vi "EQC merge1Chip.vi"(9 "EQ Leak# folder paths":path[](array[path]), 11 "ChipID":string) -> (0 "Error tick":bool, 1 "quants GOOD":u8, 2 "Merged report":string, 3 "Merged PixelReg":u32[](array[numeric]) format="%.0x")   [LabVIEW 2015, in "VIPM2.lvlib"]
uses:
  VIPM2.lvlib
panel:
  # "If X, some error while\nreading the files"
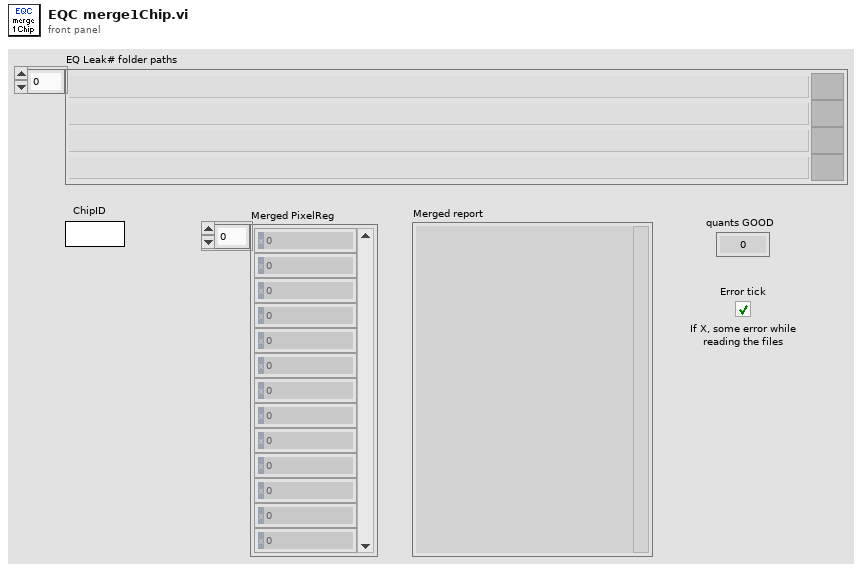
[diagram p1: front panel]
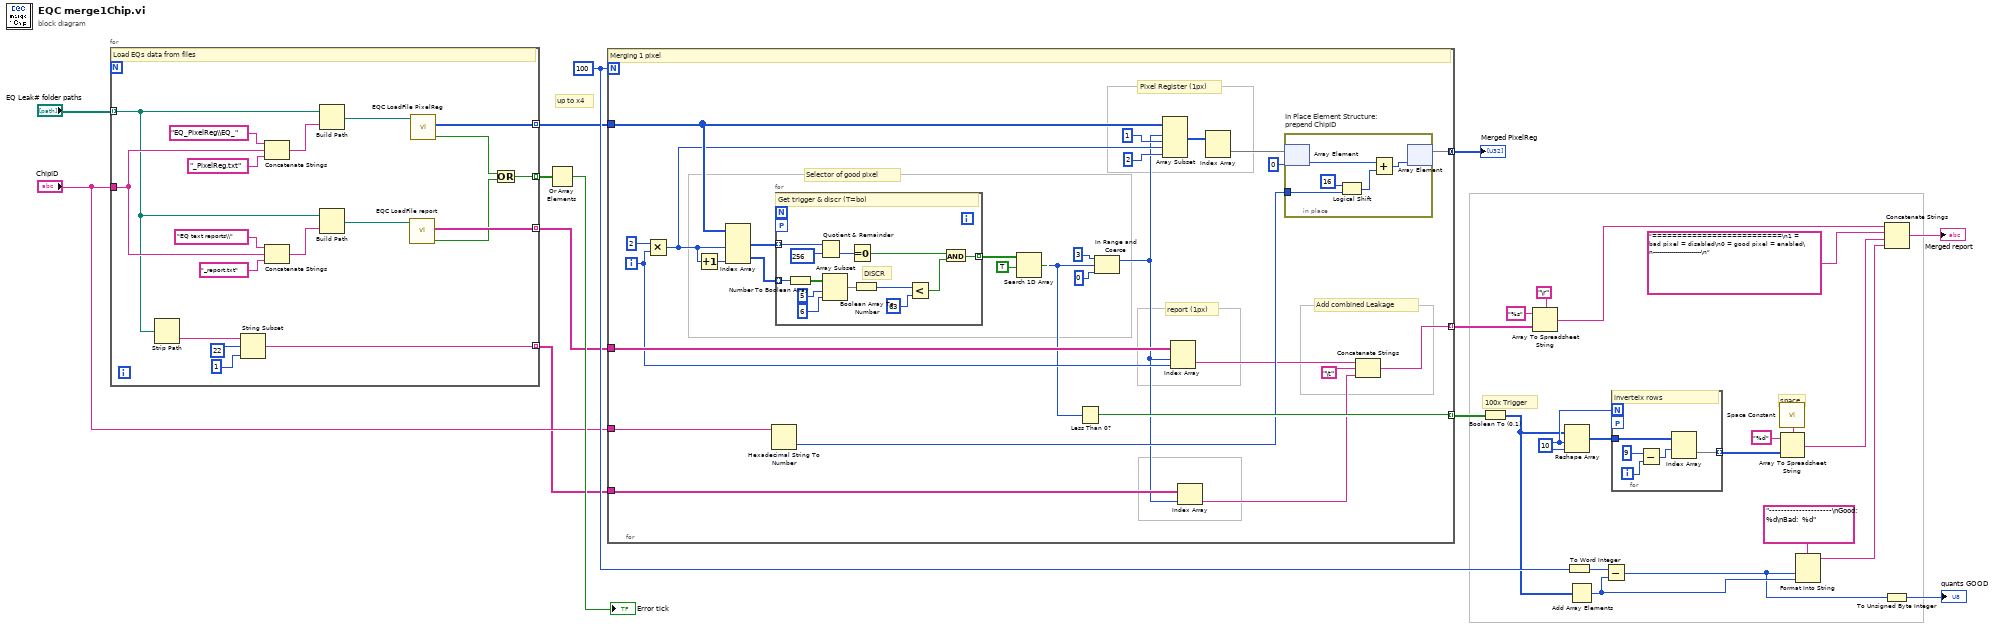
[diagram p0: block diagram]
diagram:
  w13 = 10 ("dimension size")
  w29 = 100
  # "space"
  # "100x Trigger"
  # "up to x4"
  n1 = for {
    tunnel: "EQ Leak# folder paths" -> [w34] mode=indexing
    tunnel: "ChipID" -> [w41]
    tunnel: [w39] -> w25 mode=indexing
    tunnel: [w37] -> w24 mode=indexing
    tunnel: [w35] -> w26 mode=indexing
    tunnel: [w30] -> w1 mode=indexing
    # "Load EQs data from files"
    n2 = Strip Path(path=w34) -> (name=w33:string)  [unwired: 1 out]
    n3 = String Subset(string=w33, offset (0)=22 ("offset"), length (rest)=1 ("length (rest)")) -> (substring=w30:string)
    n4 = Concatenate Strings("EQ_PixelReg\\EQ_", w41, "_PixelReg.txt") -> (w46:string)
    n5 = Concatenate Strings("EQ text reports\\", w41, "_report.txt") -> (w44:string)
    n6 = Build Path(base path=w34, name or relative path=w46) -> (appended path=w45:path)
    n7 = Build Path(base path=w34, name or relative path=w44) -> (appended path=w40:path)
    n8 = call "EQC LoadFile report.vi"("report file path"=w40) -> ("Error tick"=w36:bool, "report (1D lines)"=w37:string[])  [unwired: 9 in]
    n9 = call "EQC LoadFile PixelReg.vi"("PixelReg file path"=w45) -> ("Error tick"=w38:bool, "PixelReg (hex)"=w39:u32[])  [unwired: 9 in]
    n10 = Or(x=w38, y=w36) -> (x .or. y?=w35:bool)
  }
  n11 = Or Array Elements(Boolean array=w26) -> (logical OR=→"Error tick":bool)
  n12 = for {
    N: w29 -> [_]
    tunnel: w25 -> [w70]
    tunnel: w24 -> [w66]
    tunnel: [w61] -> w23 mode=concatenating
    tunnel: [w51] -> w22 mode=indexing
    tunnel: [w63] -> w10 mode=indexing
    tunnel: "ChipID" -> [w60]
    tunnel: w1 -> [w54]
    i -> [w65]
    # "Add combined Leakage"
    # "report (1px)"
    # "Pixel Register (1px)"
    # "Selector of good pixel"
    # "Merging 1 pixel"
    n13 = Multiply(x=2, y=w65) -> (x*y=w56:i32)
    n14 = Increment(x=w56) -> (x+1=w57:i32)
    n15 = Index Array "Index Array"(array=w70, index (col) #1=w56, index (col) #2=w57) -> (element #1=w75:u32[], element #2=w55:u32[])  [unwired: 2 in]
    n16 = Hexadecimal String To Number(string=w60) -> (number=w59:u32)  [unwired: 2 in, 1 out]
    n17 = for {
      tunnel: w75 -> [w94] mode=indexing
      tunnel: [w85] -> w74 mode=indexing
      workers-P: _ -> [_]
      tunnel: w55 -> [w91] mode=indexing
      # "DISCR"
      # "Get trigger & discr (T=bo)"
      n18 = Number To Boolean Array(number=w91) -> (Boolean array=w90:bool[])
      n19 = Quotient & Remainder(x=w94, y=u32 256) -> (floor(x/y)=w92:u32)  [unwired: 1 out]
      n20 = Array Subset(array=w90, index=5, length=6) -> (w87:bool[])
      n21 = Equal To 0?(x=w92) -> (x = 0?=w84:bool)
      n22 = Boolean Array To Number(Boolean array=w87) -> (number=w82:u32)
      n23 = Less?(x=w82, y=u32 63) -> (x < y?=w83:bool)
      n24 = And(x=w84, y=w83) -> (x .and. y?=w85:bool)
    }
    n25 = Search 1D Array(1D array=w74, element=TRUE) -> (index of element=w64:i32)  [unwired: 1 in]
    n26 = Less Than 0?(x=w64) -> (x < 0?=w63:bool)
    n27 = In Range and Coerce(upper limit=3, x=w64, lower limit=0) -> (coerced(x)=w53:i32)  [unwired: 1 out]
    n28 = Array Subset "Array Subset"(array=w70, index (row)=w53, length (row)=1 ("length"), index (col)=w56, length (col)=2 ("length")) -> (w67:u32[][])
    n29 = Index Array "Index Array"(array=w66, index (row)=w53, index (col)=w65) -> (element=w52:string)
    n30 = Index Array "Index Array"(array=w54, index=w53) -> (element=w49:string)
    n31 = Index Array "Index Array"(array=w67) -> (element=w62:u32[])  [unwired: 2 in]
    n32 = in-place "In Place Element Structure:\nprepend ChipID" {
      in-place-border: w59 -> [w81]
      n33 = in-place-array #1(w62, 0) -> (w78:u32)
      n34 = Logical Shift(y=i16 16, x=w81) -> (x << y=w79:u32)
      n35 = Add(x=w78, y=w79) -> (x+y=w77:u32)
      n36 = in-place-array #1(w77) -> (w61:u32[])  [unwired: 1 out]
    }
    n37 = Concatenate Strings "Concatenate Strings"(w52, "\t", w49) -> (w51:string)
  }
  "Merged PixelReg" <- w23
  n38 = Boolean To (0,1)(Boolean=w10) -> (0, 1=w9:i16[])
  n39 = Array To Spreadsheet String(delimiter (Tab)="\r", array=w22, 3:"%s" ("format string")) -> (spreadsheet string=w19:string)
  n40 = Reshape Array "Reshape Array"(w9, w13, w13) -> (w14:i16[][])
  n41 = To Word Integer(number=w29) -> (16bit integer=w17:i16)
  n42 = Add Array Elements(numeric array=w9) -> (sum=w15:i16)
  n43 = Subtract(x=w17, y=w15) -> (x-y=w4:i16)
  n44 = for {
    N: w13 -> [_]
    tunnel: w14 -> [w99]
    tunnel: [w95] -> w12 mode=indexing
    workers-P: _ -> [_]
    i -> [w98]
    # "inverteix rows"
    n45 = Subtract(x=9, y=w98) -> (x-y=w96:i32)
    n46 = Index Array "Index Array"(array=w99, index (row)=w96) -> (element=w95:i16[])  [unwired: 1 in]
  }
  n47 = call <vilib>:"Space Constant.vi"() -> ("String"=w5:string)
  n48 = Array To Spreadsheet String(delimiter (Tab)=w5, array=w12, 3:"%d" ("format string")) -> (spreadsheet string=w8:string)
  n49 = Format Into String(format string="---------------------\nGood: %d\nBad:  %d", w4, w15) -> (resulting string=w7:string)  [unwired: 2 in, 1 out]
  n50 = To Unsigned Byte Integer(number=w4) -> (unsigned 8bit integer=→"quants GOOD":u8)
  n51 = Concatenate Strings "Concatenate Strings"(w19, "==========================\n1 = bad pixel = disabled\n0 = good pixel = enabled\n------------------------\n", w8, w7) -> (→"Merged report":string)
